vi "zmq_proxy.vi"(4 "control":refnum<class "Socket.lvclass">, 5 "error in":errorcluster, 6 "capture":refnum<class "Socket.lvclass">, 7 "backend":refnum<class "Socket.lvclass">, 8 "frontend":refnum<class "Socket.lvclass">) -> (0 "error out":errorcluster)   [LabVIEW 2025, in "ZeroMQ.lvlib" / "Socket.lvclass"]
doc: "Starts a proxy server between the frontend and backend, with all messages passed to the capture socket, if specified. This can be used to implement a number of paradigms, such as the \"shared queue\", \"forwarder\" and \"streamer\" patterns.\n\nIf a \"control\" socket is provided, it becomes a \"steerable\" proxy.\n\nNote that this VI will not return until the host context is destroyed.\n\nDetailed API documentation: http://api.zeromq.org/3-2:zmq-proxy"
uses:
  Socket.lvclass
  Socket.lvclass/Socket.ctl
  <vilib>/Utility/error.llb/Error Cluster From Error Code.vi
  ZeroMQ.lvlib
panel:
  # "ØMQ"
  # "labview"
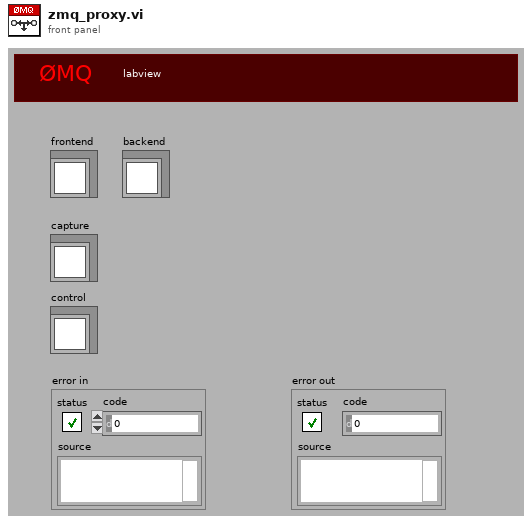
[diagram p1: front panel]
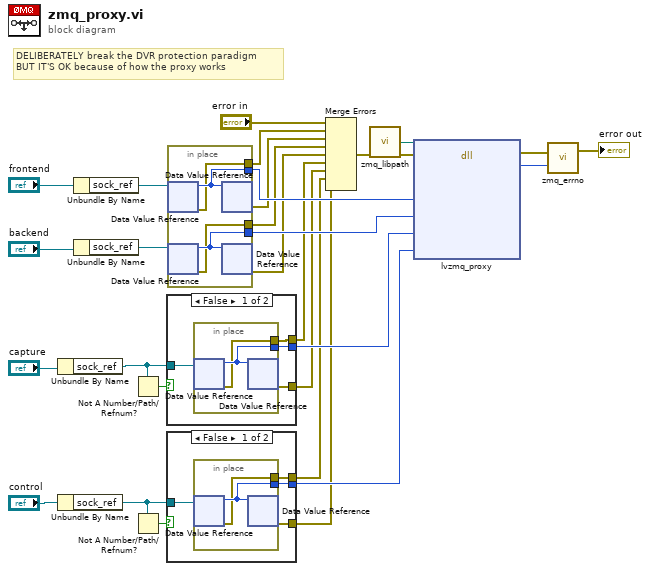
[diagram p0: block diagram]
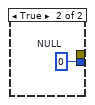
[diagram p2: hidden frame]
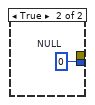
[diagram p3: hidden frame]
diagram:
  # "DELIBERATELY break the DVR protection paradigm\nBUT IT'S OK because of how the proxy works"
  n1 = Unbundle By Name("capture") -> ("sock_ref"=w7:refnum<data-value>)
  n2 = Unbundle By Name("control") -> ("sock_ref"=w9:refnum<data-value>)
  n3 = Unbundle By Name("frontend") -> ("sock_ref"=w27:refnum<data-value>)
  n4 = Unbundle By Name("backend") -> ("sock_ref"=w24:refnum<data-value>)
  n5 = Not A Number/Path/Refnum?(number/path/refnum=w7) -> (NaN/Path/Refnum?=w8:bool)
  n6 = Not A Number/Path/Refnum?(number/path/refnum=w9) -> (NaN/Path/Refnum?=w10:bool)
  n7 = case shown="False" w8 {
    tunnel: w7 -> [w32 _]
    tunnel: [w31 w35] -> w6
    tunnel: [w30 _] -> w4
    tunnel: [w29 _] -> w1
    frame False {
      n8 = in-place {
        in-place-border: [w34] -> w31
        in-place-border: [w33] -> w30
        n9 = in-place-dvr #1(w32) -> (w34:u64, w33:errorcluster)
        n10 = in-place-dvr #1(w34) -> (w29:errorcluster)  [unwired: 1 out]
      }
    }
    frame True {
      w35 = u64 0  # NULL
    }
  }
  n11 = case shown="False" w10 {
    tunnel: w9 -> [w39 _]
    tunnel: [w38 w42] -> w5
    tunnel: [w37 _] -> w3
    tunnel: [w36 _] -> w2
    frame False {
      n12 = in-place {
        in-place-border: [w41] -> w38
        in-place-border: [w40] -> w36
        n13 = in-place-dvr #2(w39) -> (w41:u64, w40:errorcluster)
        n14 = in-place-dvr #2(w41) -> (w37:errorcluster)  [unwired: 1 out]
      }
    }
    frame True {
      w42 = u64 0  # NULL
    }
  }
  n15 = in-place {
    in-place-border: [w46] -> w22
    in-place-border: [w45] -> w21
    in-place-border: [w44] -> w16
    in-place-border: [w43] -> w14
    n16 = in-place-dvr #3(w27) -> (w46:u64, w44:errorcluster)
    n17 = in-place-dvr #4(w24) -> (w45:u64, w43:errorcluster)
    n18 = in-place-dvr #3(w46) -> (w15:errorcluster)  [unwired: 1 out]
    n19 = in-place-dvr #4(w45) -> (w13:errorcluster)  [unwired: 1 out]
  }
  n20 = Merge Errors("error in", w16, w15, w14, w13, w4, w1, w2, w3) -> (w12:errorcluster)
  n21 = call "zmq_libpath.vi"() -> ("path"=w19:path)  [unwired: 1 in]
  n22 = dll-call lib="?" fn="lvzmq_proxy" ("zmq_labview.dll:lvzmq_socket")(path in=w19, error in=w12, "front"=w22, "back"=w21, "capture"=w6, "control"=w5) -> (error out=w20:errorcluster, "return type"=w18:i32)  [unwired: 7 in, 1 out]
  n23 = call "zmq_errno.vi"("retval"=w18, "error in"=w20) -> ("error out"=→"error out":errorcluster)  [unwired: 1 out]
